vi "Get Scrollbar.vi"(8 "error in (no error)":errorcluster, 11 "PanelArray in":refnum<class "PanelArray.lvclass">) -> (0 "error out":errorcluster, 2 "Scrollbar":refnum<vi>, 3 "PanelArray out":refnum<class "PanelArray.lvclass">)   [LabVIEW 2018, in "OOPanel.lvlib" / "PanelArray.lvclass"]
uses:
  PanelArray.lvclass
  PanelArray.lvclass/PanelArray.ctl
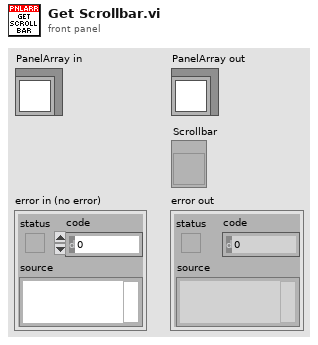
[diagram p1: front panel]
types:
  T1 = typedef "OOPanel.lvlib/PanelArray.lvclass/Ref Data.ctl" = cluster{"State":T2, "Refs":T3, "Events":T4, "Scrolling":T5, "Panels":T6}
  T2 = typedef "OOPanel.lvlib/PanelArray.lvclass/State.ctl" = cluster{"Defer Updates":bool, "Running":bool, "Dynamic Sizing":bool, "Borders":bool}
  T3 = typedef "OOPanel.lvlib/PanelArray.lvclass/Refs.ctl" = cluster{"SubPanels":refnum<vi>[], "Scrollbar":refnum<vi>, "Owning Panel":refnum<vi>}
  T4 = typedef "OOPanel.lvlib/PanelArray.lvclass/Events.ctl" = cluster{"Close":refnum<user-event>}
  T5 = typedef "OOPanel.lvlib/PanelArray.lvclass/Scrolling.ctl" = cluster{"Size":i32, "Max":i32, "Current":i32, "Top Index":i32, "Heights":i32[]}
  T6 = typedef "OOPanel.lvlib/PanelArray.lvclass/Panels.ctl" = cluster{"All":refnum<class "Panel.lvclass">[], "Visible":refnum<class "Panel.lvclass">[], "Blank":refnum<class "ArrayBlank.lvclass">}
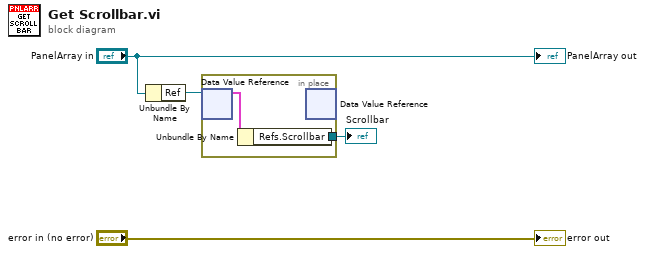
[diagram p0: block diagram]
diagram:
  n1 = Unbundle By Name("PanelArray in") -> ("Ref"=w3:refnum<data-value>)
  n2 = in-place {
    in-place-border: [w5] -> w1
    n3 = in-place-dvr #1(w3) -> (w6:T1)  [unwired: 1 out]
    n4 = Unbundle By Name(w6) -> ("Refs.Scrollbar"=w5:refnum<vi>)
    n5 = in-place-dvr #1() -> ()  [unwired: 1 in, 2 out]
  }
  "Scrollbar" <- w1
  "error out" <- "error in (no error)"
  "PanelArray out" <- "PanelArray in"
